vi "Output Actor Request Snip.vi"() -> ()   [LabVIEW 2015]
uses:
  Output Actor/Output Actor.lvclass
  Request/request.lvclass
  Request/request.lvclass/request.ctl
  <vilib>/addons/lv-msgpack/MsgPack Deserializer/Unflatten From MessagePack.vi
panel:
  out "error out":errorcluster
  in  "error in (no error)":errorcluster
  out "output_actor out":refnum<class "Output Actor.lvclass">
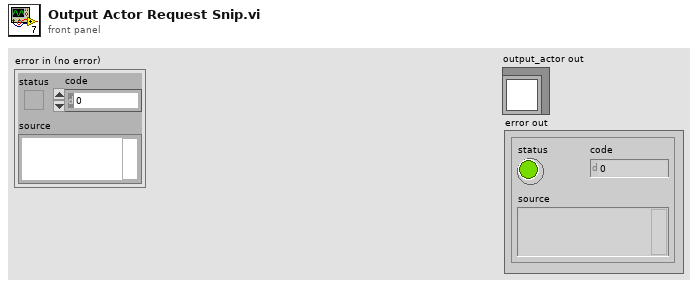
[diagram p1: front panel]
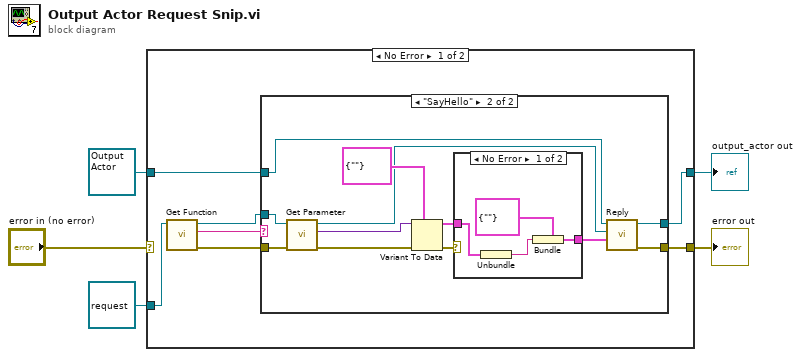
[diagram p0: block diagram]
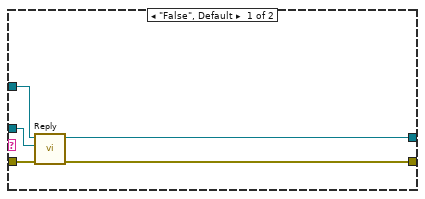
[diagram p2: hidden frame]
diagram:
  n1 = case shown="No Error" "error in (no error)" {
    selector: "error in (no error)" -> [_ w34]
    tunnel: refnum<class "request.lvclass"> refnum ("request.lvclass") -> [w12 _]
    tunnel: refnum<class "Output Actor.lvclass"> refnum ("output_actor in") -> [w10 w35]
    tunnel: [w8 w34] -> w1
    tunnel: [w7 w35] -> w2
    frame No Error {
      n2 = call "Get Function.vi"("request in"=w12) -> ("error out"=w9:errorcluster, "function"=w11:string, "request out"=w6:refnum<class "request.lvclass">)  [unwired: 8 in]
      n3 = case shown="\"SayHello\"" w11 {
        tunnel: w10 -> [w15 w29]
        tunnel: w9 -> [w17 w23]
        tunnel: [w16 w28] -> w8
        tunnel: [w14 w27] -> w7
        tunnel: w6 -> [w13 w24]
        frame "False", Default {
          n4 = call "Reply.vi"("error in (no error)"=w17, "request"=w13, "output_actor in"=w15) -> ("error out"=w16:errorcluster, "output_actor out"=w14:refnum<class "Output Actor.lvclass">)  [unwired: 7 in]
        }
        frame "SayHello" {
          n5 = call "Get Parameter.vi"("error in (no error)"=w23, "request in"=w24) -> ("error out"=w22:errorcluster, "parameter"=w20:variant, "request out"=w18:refnum<class "request.lvclass">)  [unwired: 7 in]
          n6 = Variant To Data(error in=w22, type=cluster{"Greeting":string} {"Greeting"=""}, Variant=w20) -> (data=w25:cluster{"Greeting":string}, error out=w21:errorcluster)
          n7 = case shown="No Error" w21 {
            tunnel: w25 -> [w33 _]
            tunnel: [w30 _] -> w19
            frame No Error {
              n8 = Unbundle(w33) -> ("Greeting"=w32:string)
              n9 = Bundle(cluster=cluster{"Answer":string} {"Answer"=""}, "Answer"=w32) -> (w30:cluster{"Answer":string})
            }
            frame Error {
            }
          }
          n10 = call "Reply.vi"("Result"=w19, "request"=w18, "output_actor in"=w29) -> ("error out"=w28:errorcluster, "output_actor out"=w27:refnum<class "Output Actor.lvclass">)  [unwired: 7 in]
        }
      }
    }
    frame Error {
    }
  }
  "output_actor out" <- w2
  "error out" <- w1
